vi "Sequencer List Entry Clear.vi"(8 "error in (no error)":errorcluster, 10 "Instance (1)":i32=1, 11 "VISA resource name":refnum<visa-resource-name>) -> (0 "error out":errorcluster, 3 "VISA resource name out":refnum<visa-resource-name>)   [LabVIEW 2015, in "Rohde&Schwarz CMXP GPRF.lvlib"]
doc: "Deletes all entries of the sequencer list and creates an entry with default settings.\n\nAttribute:\nRSCMXPGPRF_ATTR_SEQUENCER_LIST_ENTRY_CLEAR\n\nRemote-control command:\nSOURce:GPRF:GEN<i>:SEQuencer:LIST:ENTRy:CALL"
uses:
  <instrlib>/Rohde&Schwarz CMXP GPRF/Rohde&Schwarz CMXP GPRF.lvlib
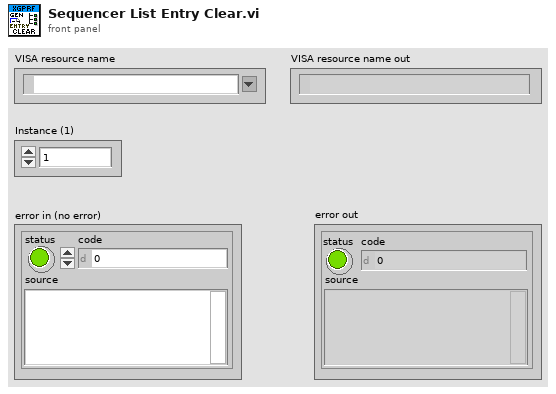
[diagram p1: front panel]
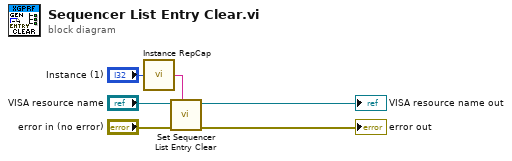
[diagram p0: block diagram]
diagram:
  n1 = call <instrlib>:"Instance RepCap.vi"("instance  in"="Instance (1)") -> ("instance out"=w1:string)
  n2 = call "Set Sequencer List Entry Clear"("Repeated Capabilities"=w1, "error in (no error)"="error in (no error)", "instrument handle"="VISA resource name") -> ("error out"=→"error out":errorcluster, "instrument handle out"=→"VISA resource name out":refnum<visa-resource-name>)  [unwired: 7 in]
